vi "get data definition.vi"(10 "channel classification":T1, 11 "RTResourceUtilitzation runtime in":refnum<class "RTResourceUtilitzation runtime.lvclass">) -> (1 "valid?":bool, 2 "index cluster":variant, 3 "RTResourceUtilitzation runtime out":refnum<class "RTResourceUtilitzation runtime.lvclass">)   [LabVIEW 2014, in "RTResourceUtilitzation runtime.lvclass"]
uses:
  RTResourceUtilitzation runtime.lvclass
  <vilib>/NI/Tag Bus Module Framework/channel/channel classification.ctl
  input user data.ctl
  output user data.ctl
  parameter user data.ctl
  result user data.ctl
  <vilib>/NI/Tag Bus Module Framework/channel/TBM channel.lvclass
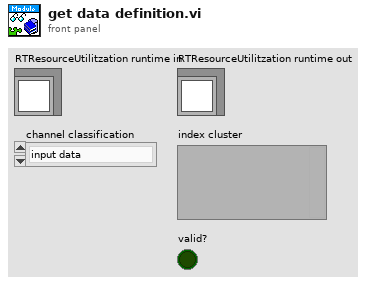
[diagram p1: front panel]
types:
  T1 = typedef "TBM channel.lvclass/channel classification.ctl" = enum16{"input data", "output data", "processing parameter", "processing result"}
  T2 = typedef "RTResourceUtilitzation runtime.lvclass/input user data.ctl" = cluster{"CPU_Usage":dbl[], "CPU_UsageTotal":dbl, "MemoryUsage":dbl, "MemoryUsagePercentage":dbl, "DiskUsage":dbl, "DiskUsagePercentage":dbl}
  T3 = typedef "RTResourceUtilitzation runtime.lvclass/output user data.ctl" = cluster{"fmwk_placeholder":i32}
  T4 = typedef "RTResourceUtilitzation runtime.lvclass/parameter user data.ctl" = cluster{"fmwk_placeholder":i32}
  T5 = typedef "RTResourceUtilitzation runtime.lvclass/result user data.ctl" = cluster{"fmwk_placeholder":i32}
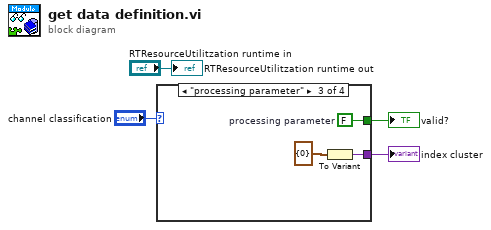
[diagram p0: block diagram]
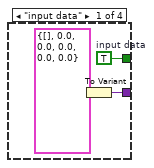
[diagram p2: hidden frame]
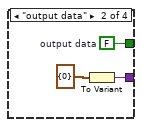
[diagram p3: hidden frame]
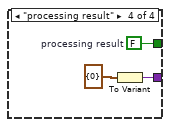
[diagram p4: hidden frame]
diagram:
  n1 = case shown="\"processing parameter\"" "channel classification" {
    tunnel: [w6 w10 w13 w16] -> w2
    tunnel: [w5 w9 w12 w15] -> w1
    frame "input data" {
      w5 = TRUE  # input data
      n2 = To Variant(anything=T2 {"CPU_Usage"=[], "CPU_UsageTotal"=0.0, "MemoryUsage"=0.0, "MemoryUsagePercentage"=0.0, "DiskUsage"=0.0, "DiskUsagePercentage"=0.0} ("Inputs from system")) -> (Variant=w6:variant)
    }
    frame "output data" {
      w9 = FALSE  # output data
      n3 = To Variant(anything=T3 {"fmwk_placeholder"=0} ("Outputs to system")) -> (Variant=w10:variant)
    }
    frame "processing parameter" {
      w12 = FALSE  # processing parameter
      n4 = To Variant(anything=T4 {"fmwk_placeholder"=0} ("Parameters to process")) -> (Variant=w13:variant)
    }
    frame "processing result" {
      w15 = FALSE  # processing result
      n5 = To Variant(anything=T5 {"fmwk_placeholder"=0} ("Results from processing")) -> (Variant=w16:variant)
    }
  }
  "index cluster" <- w2
  "valid?" <- w1
  "RTResourceUtilitzation runtime out" <- "RTResourceUtilitzation runtime in"
